vi "SensorDataUpdater.vi"   [LabVIEW 2012]
uses:
  BotStatus.vi
types:
  T1 = typedef "WPI_AnalogChannelDevRef.ctl" = cluster{"DevStatus":errorcluster, "Analog Module":T2, "Analog Channel":T3}
  T2 = typedef "FPGA_TypedefAnalogModule.ctl" = enum16{"Analog Module 1", "Analog Module 2"}
  T3 = typedef "FPGA_AIChannel.ctl" = enum8{"AI 1", "AI 2", "AI 3", "AI 4", "AI 5", "AI 6", "AI 7", "AI 8", "Invalid"}
  T4 = cluster{"Middle":bool, "InCannon":bool, "InFlipper":bool, "FlipperAtPlace":bool, "Bottom":bool, "FrisbeeDirection":bool}
  T5 = typedef "WPI_DigitalInputDevRef.ctl" = cluster{"DevStatus":errorcluster, "DIO Channel":T6, "Digital Module":T7}
  T6 = typedef "FPGA_DIOChannel.ctl" = enum8{"DIO 1", "DIO 2", "DIO 3", "DIO 4", "DIO 5", "DIO 6", "DIO 7", "DIO 8", "DIO 9", "DIO 10", "DIO 11", "DIO 12", "DIO 13", "DIO 14", "Invalid"}
  T7 = typedef "FPGA_TypedefDigitalModule.ctl" = enum16{"Digital Module 1", "Digital Module 2"}
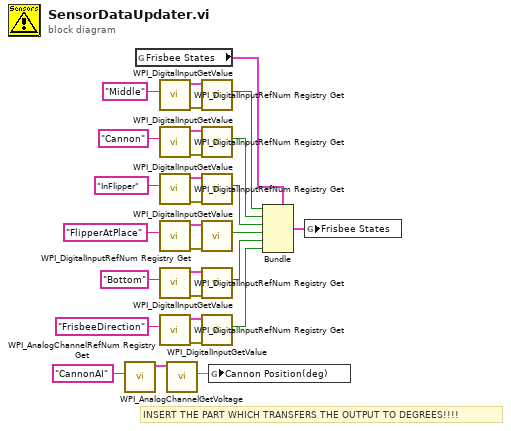
[diagram p0: block diagram]
diagram:
  # "INSERT THE PART WHICH TRANSFERS THE OUTPUT TO DEGREES!!!!"
  n1 = call <vilib>:"WPI_AnalogChannelRefNum Registry Get.vi"("refnum name"="CannonAI") -> ("AIDeviceRef"=w2:T1)  [unwired: 9 in, 1 out]
  n2 = global read "BotStatus.vi" "Frisbee States"() -> (w14:T4)
  n3 = call <vilib>:"WPI_DigitalInputRefNum Registry Get.vi"("refnum name"="Middle") -> ("error out"=w15:errorcluster, "DigitalInputDevRef"=w16:T5)  [unwired: 9 in]
  n4 = call <vilib>:"WPI_DigitalInputRefNum Registry Get.vi"("refnum name"="Cannon") -> ("error out"=w22:errorcluster, "DigitalInputDevRef"=w21:T5)  [unwired: 9 in]
  n5 = call <vilib>:"WPI_DigitalInputRefNum Registry Get.vi"("refnum name"="InFlipper") -> ("error out"=w20:errorcluster, "DigitalInputDevRef"=w19:T5)  [unwired: 9 in]
  n6 = call <vilib>:"WPI_DigitalInputRefNum Registry Get.vi"("refnum name"="FlipperAtPlace") -> ("error out"=w7:errorcluster, "DigitalInputDevRef"=w8:T5)  [unwired: 9 in]
  n7 = call <vilib>:"WPI_DigitalInputRefNum Registry Get.vi"("refnum name"="Bottom") -> ("error out"=w24:errorcluster, "DigitalInputDevRef"=w23:T5)  [unwired: 9 in]
  n8 = call <vilib>:"WPI_DigitalInputRefNum Registry Get.vi"("refnum name"="FrisbeeDirection") -> ("error out"=w18:errorcluster, "DigitalInputDevRef"=w17:T5)  [unwired: 9 in]
  n9 = call <vilib>:"WPI_AnalogChannelGetVoltage.vi"("AIDeviceRef"=w2) -> ("Voltage"=w1:dbl)  [unwired: 8 in, 2 out]
  n10 = call <vilib>:"WPI_DigitalInputGetValue.vi"("error in (no error)"=w15, "DigitalInputDevRef"=w16) -> ("Value"=w11:bool)  [unwired: 7 in, 2 out]
  n11 = call <vilib>:"WPI_DigitalInputGetValue.vi"("error in (no error)"=w22, "DigitalInputDevRef"=w21) -> ("Value"=w10:bool)  [unwired: 7 in, 2 out]
  n12 = call <vilib>:"WPI_DigitalInputGetValue.vi"("error in (no error)"=w20, "DigitalInputDevRef"=w19) -> ("Value"=w9:bool)  [unwired: 7 in, 2 out]
  n13 = call <vilib>:"WPI_DigitalInputGetValue.vi"("error in (no error)"=w7, "DigitalInputDevRef"=w8) -> ("Value"=w5:bool)  [unwired: 7 in, 2 out]
  n14 = call <vilib>:"WPI_DigitalInputGetValue.vi"("error in (no error)"=w24, "DigitalInputDevRef"=w23) -> ("Value"=w12:bool)  [unwired: 7 in, 2 out]
  n15 = call <vilib>:"WPI_DigitalInputGetValue.vi"("error in (no error)"=w18, "DigitalInputDevRef"=w17) -> ("Value"=w4:bool)  [unwired: 7 in, 2 out]
  n16 = global write "BotStatus.vi" "Cannon Position(deg)"(w1) -> ()
  n17 = Bundle(cluster=w14, "Middle"=w11, "InCannon"=w10, "InFlipper"=w9, "FlipperAtPlace"=w5, "Bottom"=w12, "FrisbeeDirection"=w4) -> (w13:T4)
  n18 = global write "BotStatus.vi" "Frisbee States"(w13) -> ()
